vi "Consumer.vi"(8 "error in (no error)":errorcluster, 9 "Data":variant, 10 "Case ID":string, 11 "Scheduler in":refnum<class "Scheduler.lvclass">) -> (0 "error out":errorcluster, 3 "Scheduler out":refnum<class "Scheduler.lvclass">)   [LabVIEW 2020, in "TALOS.lvlib" / "Scheduler.lvlib" / "Scheduler.lvclass"]
uses:
  Scheduler.lvclass
  C:/LabVIEW Code/TALOS/talos/Father of all uServices/Father of all uServices/Father of all uServices.lvclass
  Scheduler Consumer Case Selector.ctl
  Father of all uServices/Father of all uServices/Father of all uServices.lvclass/Father of all uServices.ctl
  Ancestor/Ancestor/Ancestor.lvclass/Ancestor.ctl
  Add RUN Output Data Packet.ctl
  Run Utilities/Schedule Block/Schedule Block.lvclass
  Scheduler.lvclass/Scheduler.ctl
  Run Utilities/Sequence of SBlocks/Sequence of SBlocks.lvclass
  Run Utilities/TypeDefs/Synchronize FPGA Cluster.ctl
  Run Utilities/TypeDefs/Messages/Schedule Message - Standard.ctl
  Run Utilities/Schedule/Schedule.lvclass
  Run Utilities/TypeDefs/Messages/Schedule Message - Parallel.ctl
  Guardian/Guardian Messages/Message to uService Msg/Message to uService Msg.lvclass/Message to uService Msg.ctl
  Father of all uServices/Father of all uServices Messages/Consumer Msg/Consumer Msg.lvclass/Consumer Msg.ctl
  Selection.ctl
  cc9169f9-c1ee-4f38-a286-790ff9248fc5.vi
  Support VIs/Generate Error.vi
  Guardian/Guardian Messages/Message to uService Msg/Send Message to uService.vi
  FGV/Error Memory/Get Error Description.vi
  Support VIs/Get PC name.vi
  Ancestor/Ancestor/Read ID.vi
  Support VIs/Get Class Name.vi
  FGV/Error Memory/Error Memory Core.vi
  <vilib>/AdvancedString/Delimited String to 1D String Array.vi
  Support VIs/Circus Root Path.vi
  FGV/Error Memory/Error Crt Lvl checker.vi
  FGV/Error Memory/Error Memory Core.vi/40c8088d-b597-4017-91af-faa98e00292e.vi
  FGV/Error Memory/Error Memory Core.vi/d4a3ab98-063c-4e44-b43d-fbdcfe6c2be2.vi
  Father of all uServices/Father of all uServices/Father of all uServices.lvclass
  C:/LabVIEW Code/TALOS/builds/Actor Framework PPL/Actor Framework.lvlibp/1abvi3w/vi.lib/ActorFramework/Actor/Actor.lvclass
  Support VIs/Global Memory.vi
  <vilib>/Utility/LVClass/Get LV Class Name.vi
  Support VIs/Is in Packed Library.vi
  Support VIs/TALOS Root path.vi
  Support VIs/Read CSV worksheet.vi
  Support VIs/Global Constants.vi
  <vilib>/Utility/error.llb/General Error Handler.vi
  Support VIs/Error Log.vi
  Add RUN Window.vi
  Father of all uServices/Father of all uServices/Children Methods/Get GUI Item Value - Variant.vi
  builds/Actor Framework PPL/Actor Framework.lvlibp/1abvi3w/vi.lib/ActorFramework/Actor/Read Caller Enqueuer.vi
  builds/Actor Framework PPL/Actor Framework.lvlibp/1abvi3w/vi.lib/ActorFramework/Message Enqueuer/Enqueue.vi
  builds/Actor Framework PPL/Actor Framework.lvlibp/1abvi3w/vi.lib/ActorFramework/Actor/Read Self Enqueuer.vi
  <userlib>/_OpenG.lib/lvdata/lvdata.llb/Get Strings from Enum__ogtk.vi
  Ancestor/Ancestor/Ancestor.lvclass
  <vilib>/Comparison/Equal/Equal Functor/Equal Functor.lvclass
  Guardian/Guardian Messages/Message to uService Msg/Message to uService Msg.lvclass
  Father of all uServices/Father of all uServices Messages/Consumer Msg/Consumer Msg.lvclass
  Scheduler.lvlib
  C:/LabVIEW Code/TALOS/talos/Ancestor/Ancestor/Ancestor.lvclass
  C:/LabVIEW Code/TALOS/talos/Internal uServices/CIRCUS uServices/Scheduler/Scheduler.lvclass
  Run Utilities/Run Utilities.lvlib
  TALOS.lvlib
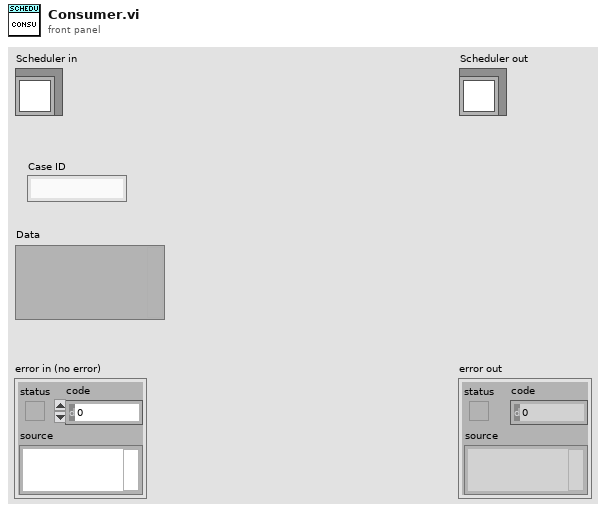
[diagram p1: front panel]
types:
  T1 = typedef "TALOS.lvlib/Scheduler.lvlib/Scheduler.lvclass/Scheduler Consumer Case Selector.ctl" = enum16{"Add SBlock", "Update GUI", "Move SBlock", "Select SBlock", "Update Cont.", "Load", "Save", "Reset", "Send to Tamer", "Edit SBlock", "Duplicate SBlock", "Delete SBlock", "Update SBlock", "Init", "Split/Combine Schedules", "Reschedule", "Load Parameters"}
  T2 = enum8{"Enabled", "Disabled", "Disabled and Grayed Out"}
  T3 = typedef "TALOS.lvlib/Scheduler.lvlib/Scheduler.lvclass/Add RUN Output Data Packet.ctl" = cluster{"Index":i32, "Schedule Block":refnum<class "Schedule Block.lvclass">}
  T4 = enum32{"Invalid", "Standard", "Closed", "Hidden", "Minimized", "Maximized"}
  T5 = typedef "TALOS.lvlib/Run Utilities.lvlib/Schedule Message - Standard.ctl" = cluster{"Schedules":refnum<class "Schedule.lvclass">[]}
  T6 = typedef "TALOS.lvlib/Run Utilities.lvlib/Schedule Message - Parallel.ctl" = cluster{"Schedules":refnum<class "Schedule.lvclass">[], "Synchronised":T7[]}
  T7 = typedef "TALOS.lvlib/Run Utilities.lvlib/Synchronize FPGA Cluster.ctl" = cluster{"Status":bool, "FPGA Name":string}
  T8 = typedef "TALOS.lvlib/Scheduler.lvlib/Scheduler.lvclass/Selection.ctl" = cluster{"Row":i32, "Column":i32}
  T9 = typedef "TALOS.lvlib/Run Utilities.lvlib/Sequence of SBlocks.lvclass/Sequence of SBlcoks - GUI.ctl" = cluster{"Total number of scripts":i32, "Time":string, "Sequence of SBlocks":T10[], "Continuous":bool}
  T10 = typedef "TALOS.lvlib/Run Utilities.lvlib/Schedule Block.lvclass/Schedule Block - simplified GUI.ctl" = cluster{"Bcg Color":u32, "Index":i32, "No. of runs":i32, "Script name":string, "FPGA name":string, "Parameters":string, "Repetitions":i32}
  T11 = cluster{"SBlock Index":i32, "Sequence Index":i32}
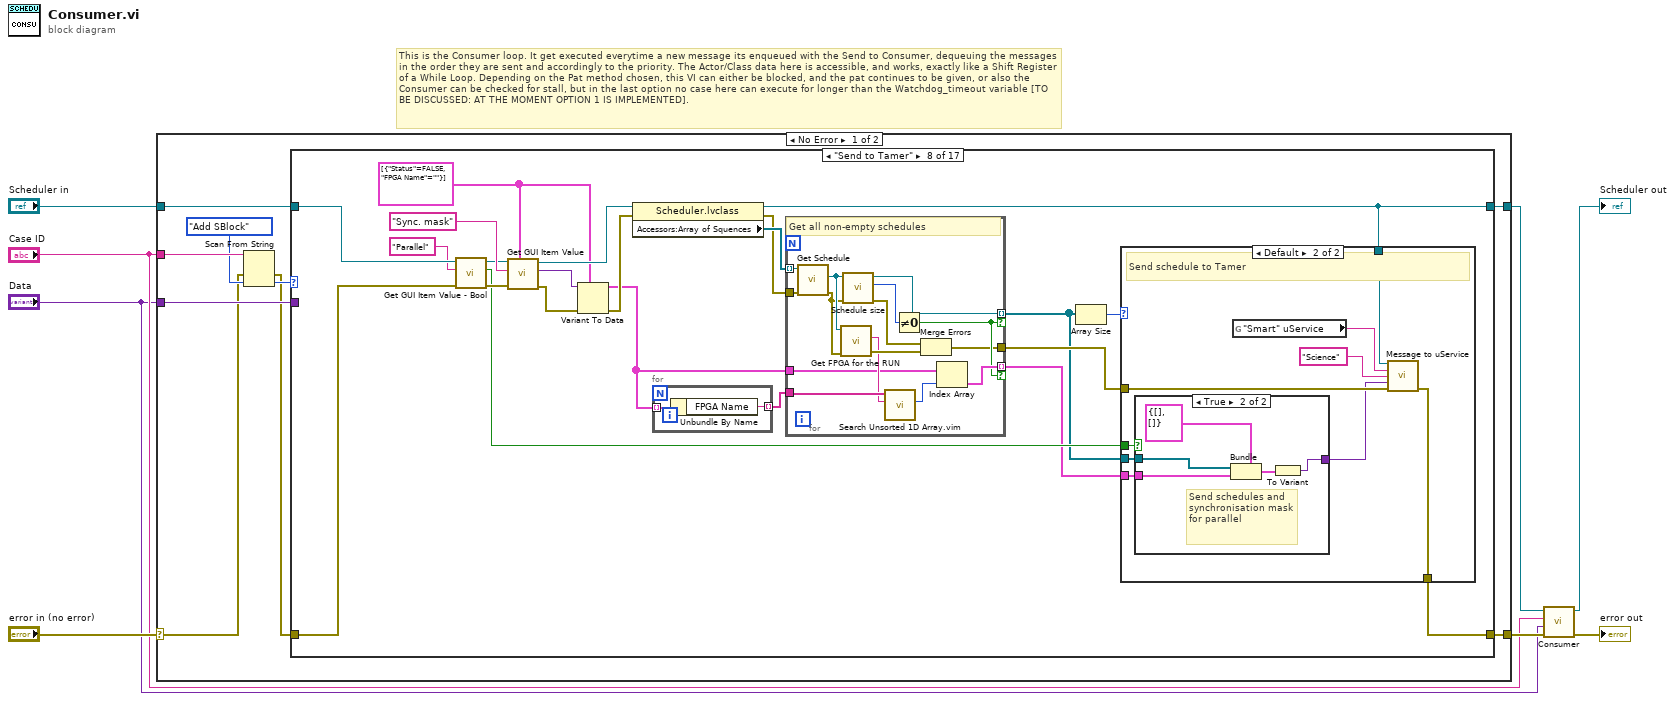
[diagram p0: block diagram]
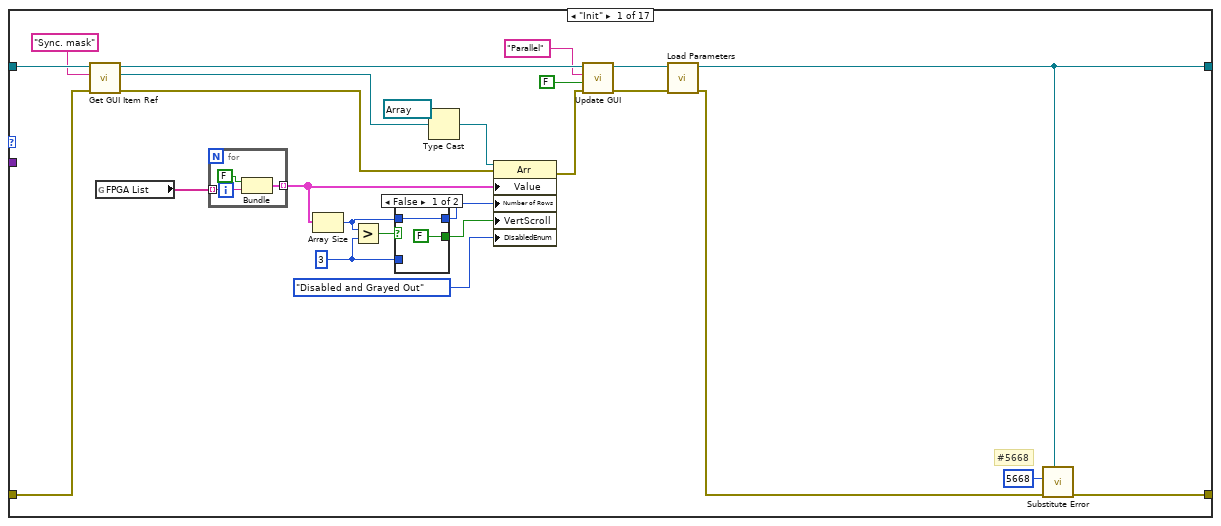
[diagram p2: hidden frame]
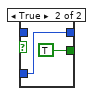
[diagram p3: hidden frame]
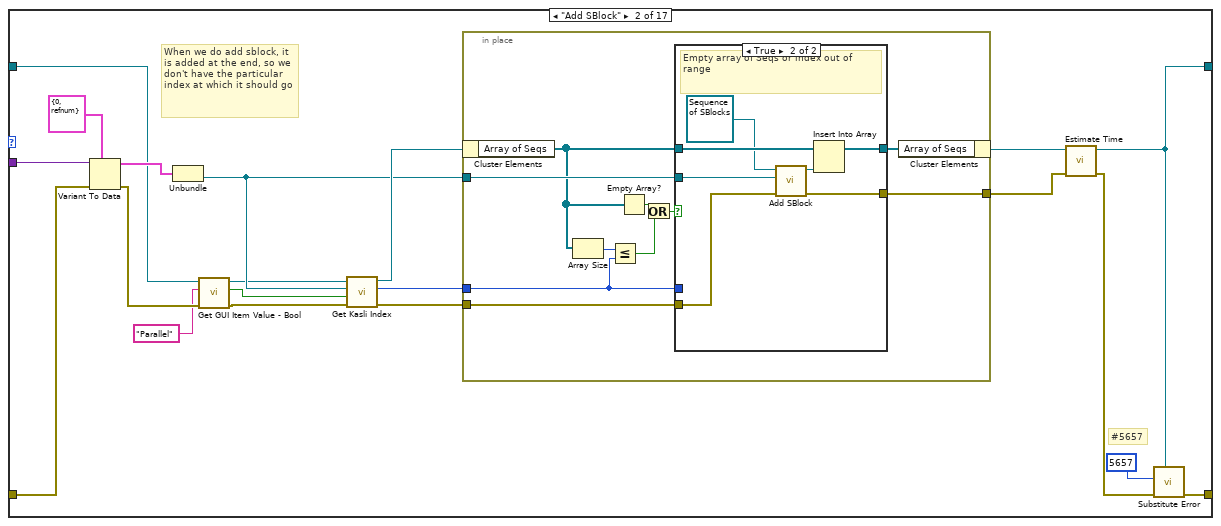
[diagram p4: hidden frame]
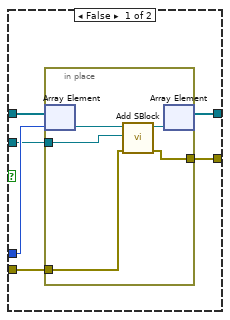
[diagram p5: hidden frame]
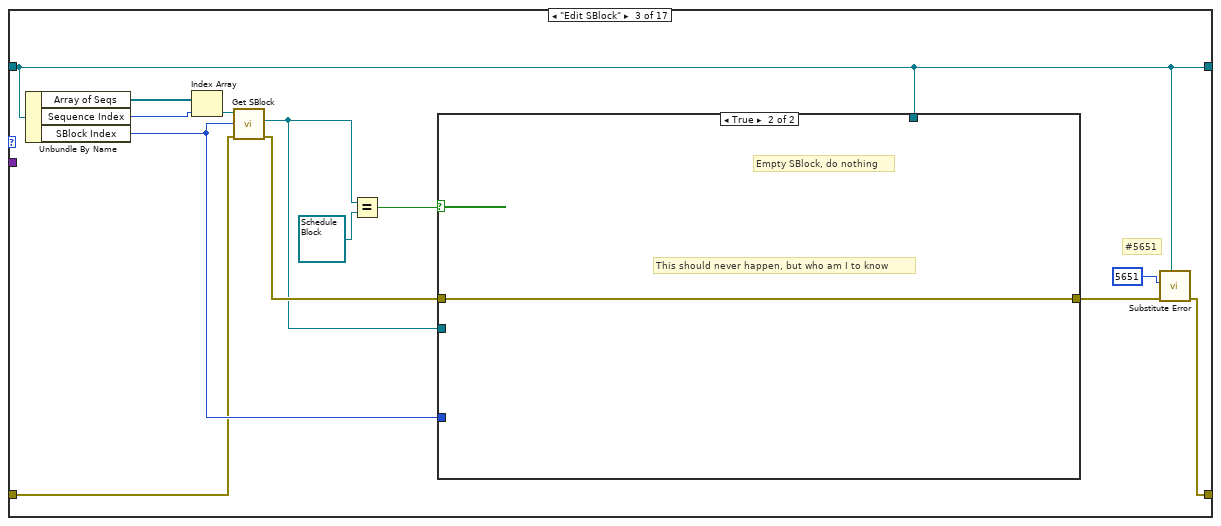
[diagram p6: hidden frame]
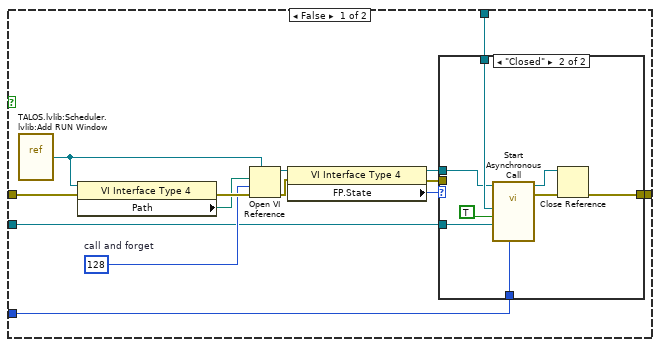
[diagram p7: hidden frame]
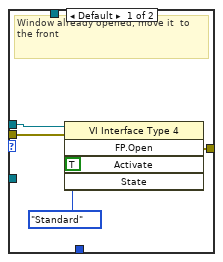
[diagram p8: hidden frame]
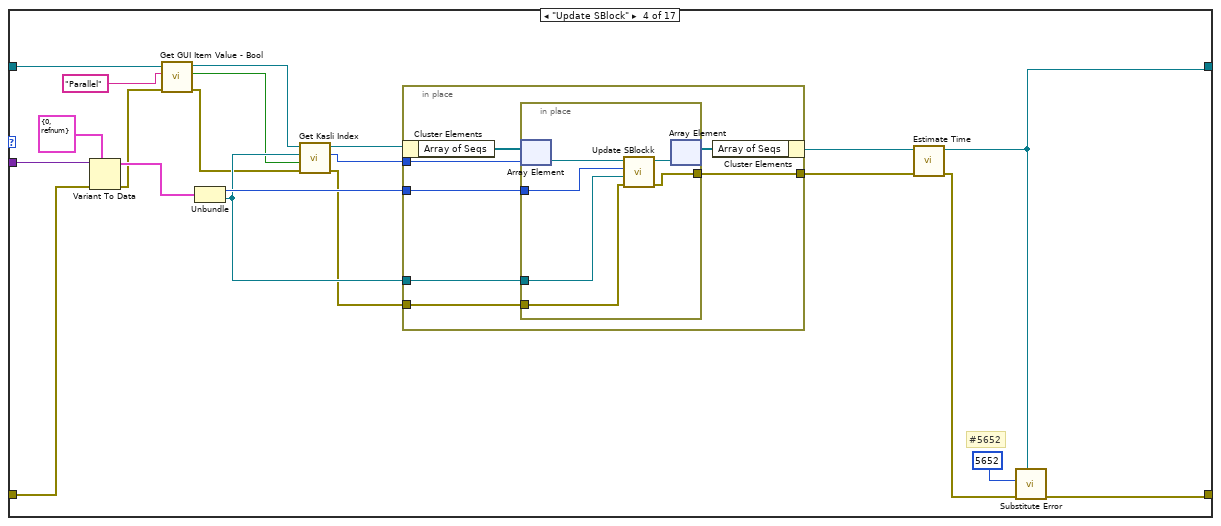
[diagram p9: hidden frame]
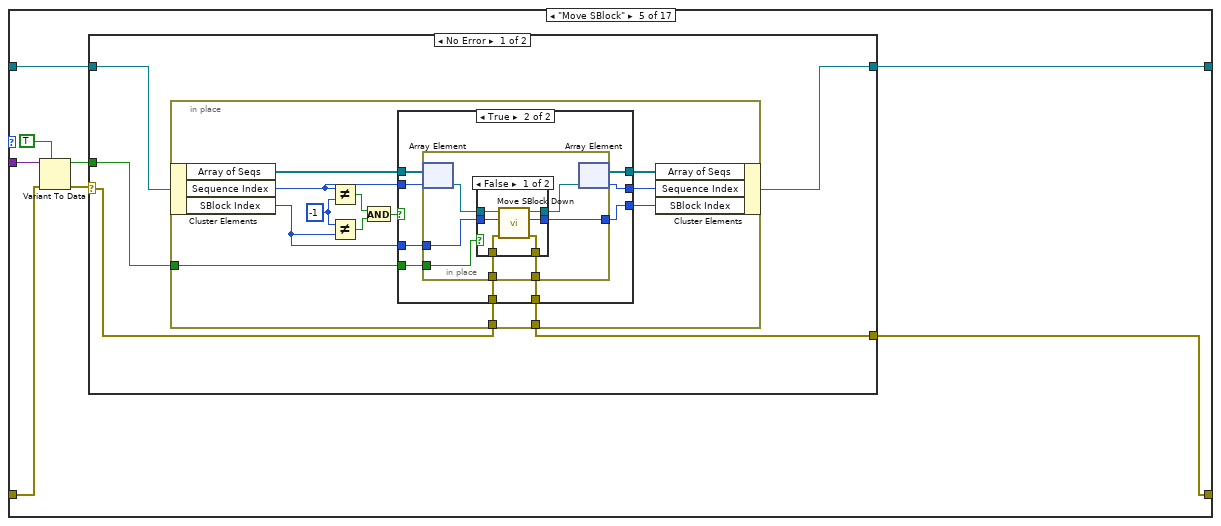
[diagram p10: hidden frame]
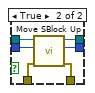
[diagram p12: hidden frame]
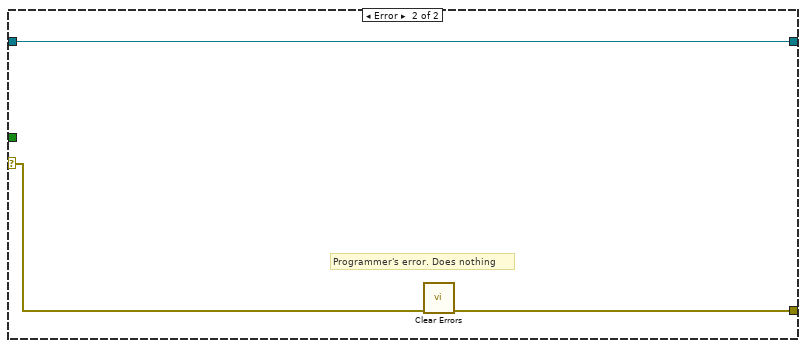
[diagram p13: hidden frame]
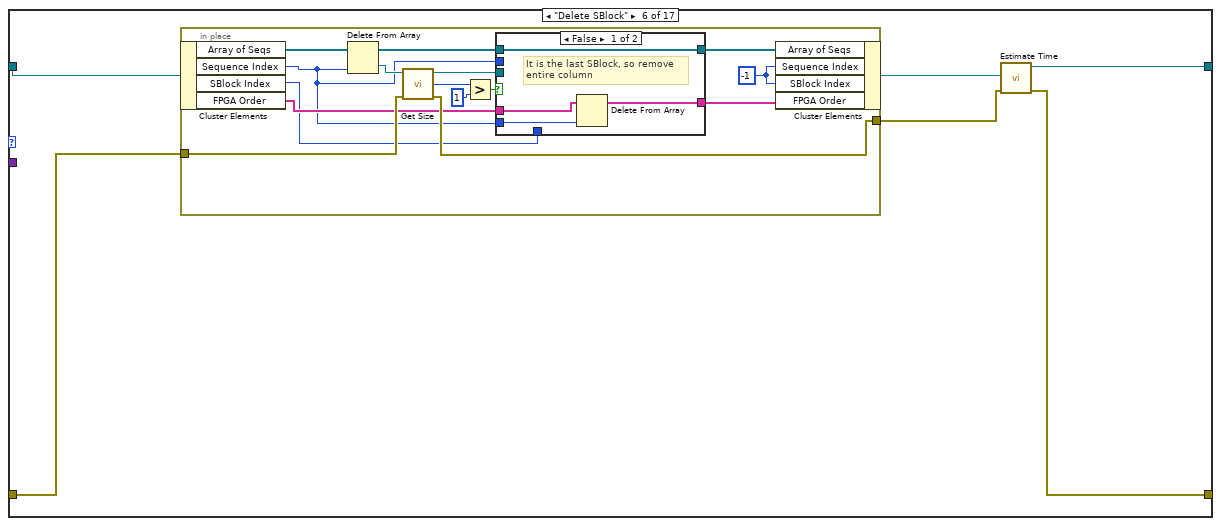
[diagram p14: hidden frame]
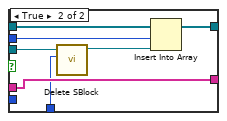
[diagram p15: hidden frame]
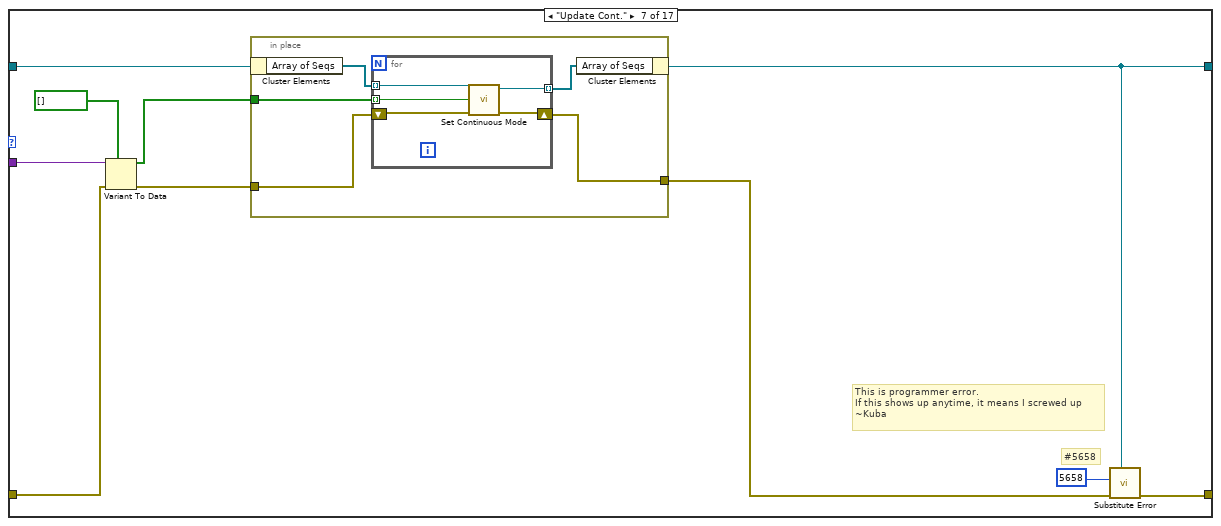
[diagram p16: hidden frame]
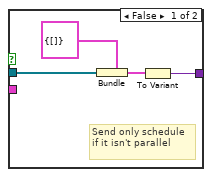
[diagram p18: hidden frame]
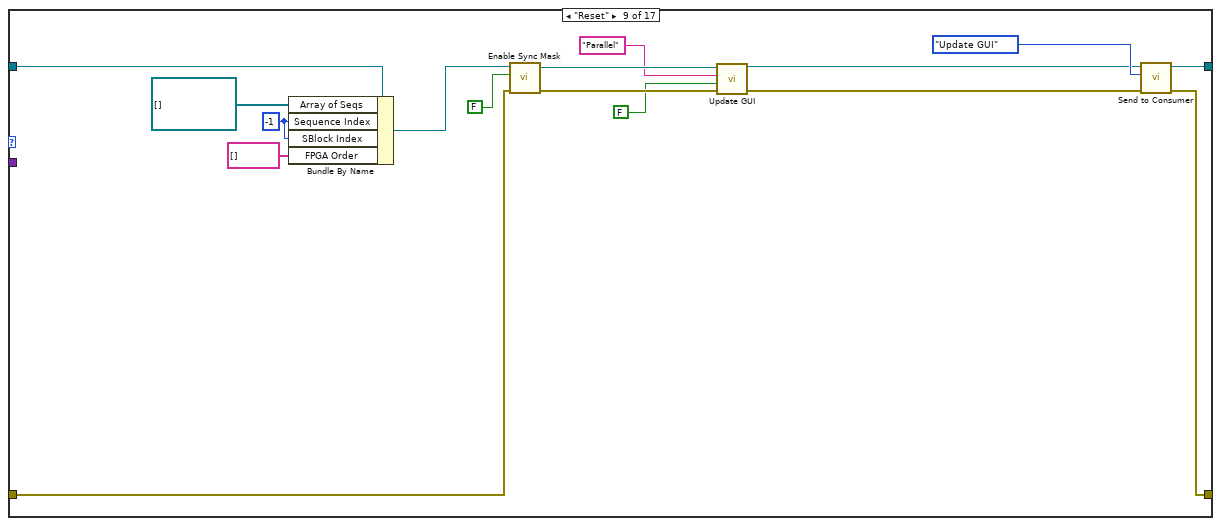
[diagram p19: hidden frame]
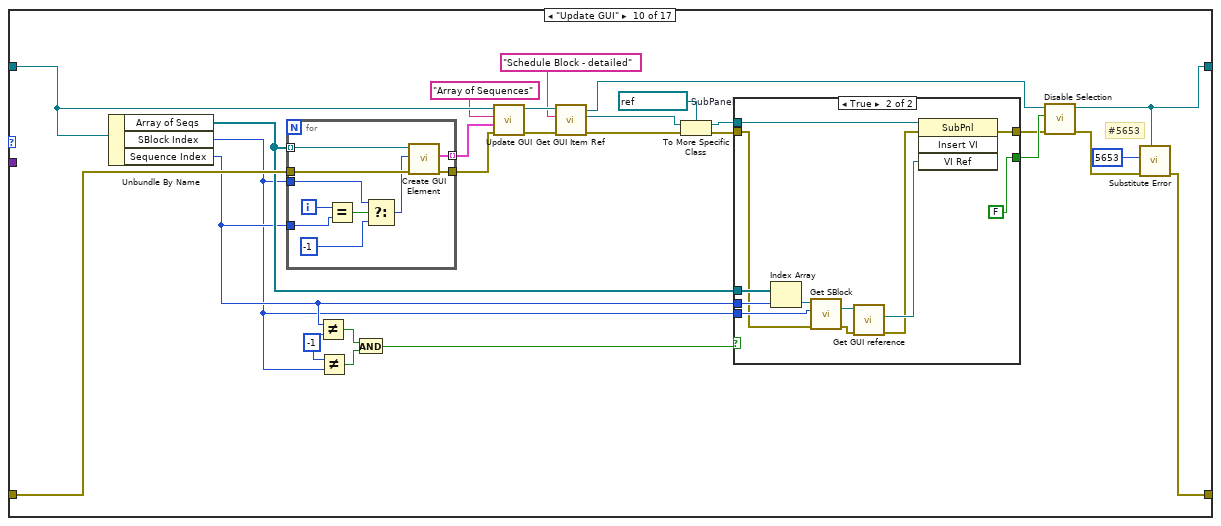
[diagram p20: hidden frame]
diagram:
  # "This is the Consumer loop. It get executed everytime a new message its enqueued with the Send to Consumer, dequeuing the messages in the order they are sent and accordingly to the priority. The Actor/Class data here is accessible, and works, exactly like a Shift Register of a While Loop. Depending on the Pat method chosen, this VI can either be blocked, and the pat continues to be given, or also the Consumer can be checked for stall, but in the last option no case here can execute for longer than the Watchdog_timeout variable [TO BE DISCUSSED: AT THE MOMENT OPTION 1 IS IMPLEMENTED]."
  n1 = case shown="No Error" "error in (no error)" {
    selector: "error in (no error)" -> [w11 w602]
    tunnel: [w10 w603] -> w3
    tunnel: "Scheduler in" -> [w17 w603]
    tunnel: [w15 w602] -> w6
    tunnel: "Case ID" -> [w14 _]
    tunnel: "Data" -> [w16 _]
    frame No Error {
      n2 = Scan From String(input string=w14, error in=w11, default 1=Scheduler_Consumer_Case_Selector."Add SBlock" ("Consumer Case Selector")) -> (error out=w9:errorcluster, output 1=w12:T1)  [unwired: 2 in, 2 out]
      n3 = case shown="\"Send to Tamer\"" w12 {
        tunnel: w17 -> [w35 w55 w108 w143 w180 w239 w275 w301 w350 w384 w416 w468 w496 w519 w565 w595 w600]
        tunnel: w16 -> [_ w69 _ w159 w178 _ w274 _ _ _ w414 w467 _ w518 w567 w597 _]
        tunnel: [w20 w61 w110 w150 w173 w235 w270 w306 w358 w386 w418 w470 w490 w511 w564 w588 w598] -> w15
        tunnel: w9 -> [w34 w66 w103 w155 w174 w238 w273 w300 w347 w383 w413 w466 w497 w516 w566 w592 w601]
        tunnel: [w19 w58 w108 w147 w179 w236 w269 w305 w359 w373 w417 w469 w491 w515 w562 w589 w599] -> w10
        frame "Init" {
          w37 = 3 ("y")
          # "#5668"
          n4 = call "Get GUI Item Ref.vi"("error in (no error)"=w34, "FP Item Name"="Sync. mask", "uService Template in"=w35) -> ("error out"=w29:errorcluster, "Ctl Refnum"=w33:refnum<vi>, "uService Template out"=w28:refnum<class "Scheduler.lvclass">)  [unwired: 6 in]
          n5 = global read "Global Memory.vi" "FPGA List"() -> (w22:string[])
          n6 = for {
            tunnel: w22 -> [w48] mode=indexing
            tunnel: [w47] -> w36 mode=indexing
            n7 = Bundle(FALSE, "AEgIS PCs List"=w48) -> (w47:cluster{bool, "AEgIS PCs List":string})  [unwired: 1 in]
          }
          n8 = Array Size(array=w36) -> (size(s)=w39:i32)
          n9 = Greater?(x=w39, y=w37) -> (0:w42:bool)
          n10 = case shown="False" w42 {
            tunnel: [w43 w45] -> w41
            tunnel: [FALSE TRUE] -> w40
            tunnel: w39 -> [w43 _]
            tunnel: w37 -> [_ w45]
            frame False {
            }
            frame True {
            }
          }
          n11 = Type Cast(type=refnum<vi> refnum ("reference"), x=w33) -> (*(type *) &x=w31:refnum<vi>)
          n12 = property class="Arr"(reference=w31, error in=w29, "Value"=w36, "Number of Rows"=w41, "VertScroll"=w40, "DisabledEnum"=T2."Disabled and Grayed Out" ("Disabled")) -> (error out=w27:errorcluster)  [unwired: 1 out]
          n13 = call "Update GUI.vi"("error in (no error)"=w27, "Data"=FALSE, "GUI Item Name"="Parallel", "uService Template in"=w28) -> ("error out"=w24:errorcluster, "uService Template out"=w23:refnum<class "Scheduler.lvclass">)  [unwired: 6 in]
          n14 = call-dynamic "Load Parameters.vi"("error in (no error)"=w24, "Scheduler in"=w23) -> ("error out"=w21:errorcluster, "Scheduler out"=w19:refnum<class "Scheduler.lvclass">)  [unwired: 8 in]
          n15 = call "Substitute Error.vi"("LabVIEW Object"=w19, "error in (no error)"=w21, "Error Code"=5668) -> ("error out"=w20:errorcluster)  [unwired: 8 in]
        }
        frame "Add SBlock" {
          # "When we do add sblock, it is added at the end, so we don't have the particular index at which it should go"
          # "#5657"
          n16 = Variant To Data(error in=w66, type=T3 {"Index"=0, "Schedule Block"=refnum} ("Cluster"), Variant=w69) -> (data=w67:T3, error out=w54:errorcluster)
          n17 = Unbundle(w67) -> ("Schedule Block"=w62:refnum<class "Schedule Block.lvclass">)  [unwired: 1 out]
          n18 = call "Get GUI Item Value - Bool.vi"("error in (no error)"=w54, "FP Item Name"="Parallel", "uService Template in"=w55) -> ("error out"=w53:errorcluster, "Value"=w51:bool, "uService Template out"=w52:refnum<class "Scheduler.lvclass">)  [unwired: 6 in]
          n19 = call-dynamic "Get Kasli Index.vi"("error in (no error)"=w53, "Parallel?"=w51, "Schedule Block"=w62, "Scheduler in"=w52) -> ("error out"=w63:errorcluster, "Index"=w64:i32, "Scheduler out"=w65:refnum<class "Scheduler.lvclass">)  [unwired: 5 in]
          n20 = in-place {
            in-place-border: w64 -> [w73]
            in-place-border: w62 -> [w79]
            in-place-border: w63 -> [w77]
            in-place-border: [w76] -> w56
            n21 = in-place-cluster #1(w65) -> ("Array of Seqs"=w71:refnum<class "Sequence of SBlocks.lvclass">[])
            n22 = Array Size(array=w71) -> (size(s)=w74:i32)
            n23 = Less Or Equal?(x=w74, y=w73) -> (x <= y?=w72:bool)
            n24 = Empty Array?(array=w71) -> (empty?=w75:bool)
            n25 = Or(x=w75, y=w72) -> (x .or. y?=w70:bool)
            n26 = case shown="True" w70 {
              tunnel: w73 -> [w85 _]
              tunnel: w71 -> [w84 w97]
              tunnel: w79 -> [w83 w94]
              tunnel: [w82 w96] -> w78
              tunnel: w77 -> [w81 w92]
              tunnel: [w80 w91] -> w76
              frame False {
                n27 = in-place {
                  in-place-border: w83 -> [w87]
                  in-place-border: w81 -> [w88]
                  in-place-border: [w86] -> w80
                  n28 = in-place-array #2(w84, w85) -> (w90:refnum<class "Sequence of SBlocks.lvclass">)
                  n29 = call-dynamic "Add SBlock.vi"("error in (no error)"=w88, "new SBlock"=w87, "Sequence of SBlocks in"=w90) -> ("error out"=w86:errorcluster, "Sequence of SBlocks out"=w89:refnum<class "Sequence of SBlocks.lvclass">)  [unwired: 7 in]
                  n30 = in-place-array #2(w89) -> (w82:refnum<class "Sequence of SBlocks.lvclass">[])  [unwired: 1 out]
                }
              }
              frame True {
                # "Empty array of Seqs or index out of range"
                n31 = call-dynamic "Add SBlock.vi"("error in (no error)"=w92, "new SBlock"=w94, "Sequence of SBlocks in"=refnum<class "Sequence of SBlocks.lvclass"> refnum ("new element/subarray")) -> ("error out"=w91:errorcluster, "Sequence of SBlocks out"=w93:refnum<class "Sequence of SBlocks.lvclass">)  [unwired: 7 in]
                n32 = Insert Into Array(array=w97, new element=w93) -> (w96:refnum<class "Sequence of SBlocks.lvclass">[])  [unwired: 1 in]
              }
            }
            n33 = in-place-cluster #1("Array of Seqs"=w78) -> (w59:refnum<class "Scheduler.lvclass">)
          }
          n34 = call-dynamic "Estimate Time.vi"("error in (no error)"=w56, "Scheduler in"=w59) -> ("error out"=w57:errorcluster, "Scheduler out"=w58:refnum<class "Scheduler.lvclass">)  [unwired: 8 in]
          n35 = call "Substitute Error.vi"("LabVIEW Object"=w58, "error in (no error)"=w57, "Error Code"=5657) -> ("error out"=w61:errorcluster)  [unwired: 8 in]
        }
        frame "Edit SBlock" {
          # "#5651"
          n36 = Unbundle By Name(w108) -> ("Array of Seqs"=w106:refnum<class "Sequence of SBlocks.lvclass">[], "Sequence Index"=w105:i32, "SBlock Index"=w104:i32)
          n37 = Index Array(array=w106, index=w105) -> (element=w102:refnum<class "Sequence of SBlocks.lvclass">)
          n38 = call-dynamic "Get SBlock.vi"("error in (no error)"=w103, "index"=w104, "Sequence of SBlocks in"=w102) -> ("error out"=w101:errorcluster, "Schedule Block"=w98:refnum<class "Schedule Block.lvclass">)  [unwired: 6 in, 1 out]
          n39 = Equal?(x=w98, y=refnum<class "Schedule Block.lvclass"> refnum) -> (x = y?=w99:bool)
          n40 = case shown="True" w99 {
            tunnel: w108 -> [w123 _]
            tunnel: [w122 w138] -> w107
            tunnel: w101 -> [w121 w138]
            tunnel: w104 -> [w120 _]
            tunnel: w98 -> [w115 _]
            frame False {
              w118 = 128  # call and forget
              n41 = vi-ref "TALOS.lvlib:Scheduler.lvlib:Add RUN Window.vi"() -> (w117:refnum<vi>)
              n42 = property class="VI Interface Type 4"(reference=w117, error in=w121) -> (error out=w124:errorcluster, "Path"=w116:path)  [unwired: 1 out]
              n43 = Open VI Reference(type specifier VI Refnum (for type only)=w117, vi path=w116, options=w118, error in (no error)=w124) -> (vi reference=w119:refnum<vi>, error out=w114:errorcluster)  [unwired: 2 in]
              n44 = property class="VI Interface Type 4"(reference=w119, error in=w114) -> (reference out=w112:refnum<vi>, error out=w111:errorcluster, "FP.State"=w113:T4)
              n45 = case shown="\"Closed\"" w113 {
                tunnel: w123 -> [_ w137]
                tunnel: [w126 w136] -> w122
                tunnel: w120 -> [_ w135]
                tunnel: w115 -> [_ w131]
                tunnel: w112 -> [w125 w130]
                tunnel: w111 -> [w127 _]
                frame Default {
                  # "Window already opened, move it  to the front"
                  n46 = invoke class="VI Interface Type 4" method="FP.Open"(reference=w125, error in=w127, "Activate"=TRUE ("Activate?"), "State"=T4."Standard") -> (error out=w126:errorcluster)  [unwired: 1 in, 4 out]
                }
                frame "Closed" {
                  n47 = call-by-ref "Start Asynchronous Call"(reference=w130, "Index"=w135, "Schedule Block"=w131, "Modify"=TRUE, "Scheduler in"=w137) -> (reference out=w133:refnum<vi>, error out=w134:errorcluster)  [unwired: 7 in, 2 out]
                  n48 = Close Reference(reference=w133, error in (no error)=w134) -> (error out=w136:errorcluster)
                }
              }
            }
            frame True {
              # "This should never happen, but who am I to know"
              # "Empty SBlock, do nothing"
            }
          }
          n49 = call "Substitute Error.vi"("LabVIEW Object"=w108, "error in (no error)"=w107, "Error Code"=5651) -> ("error out"=w110:errorcluster)  [unwired: 8 in]
        }
        frame "Update SBlock" {
          # "#5652"
          n50 = Variant To Data(error in=w155, type=T3 {"Index"=0, "Schedule Block"=refnum} ("Cluster"), Variant=w159) -> (data=w157:T3, error out=w141:errorcluster)
          n51 = call "Get GUI Item Value - Bool.vi"("error in (no error)"=w141, "FP Item Name"="Parallel", "uService Template in"=w143) -> ("error out"=w140:errorcluster, "Value"=w139:bool, "uService Template out"=w142:refnum<class "Scheduler.lvclass">)  [unwired: 6 in]
          n52 = Unbundle(w157) -> ("Index"=w156:i32, "Schedule Block"=w152:refnum<class "Schedule Block.lvclass">)
          n53 = call-dynamic "Get Kasli Index.vi"("error in (no error)"=w140, "Parallel?"=w139, "Schedule Block"=w152, "Scheduler in"=w142) -> ("error out"=w151:errorcluster, "Index"=w153:i32, "Scheduler out"=w154:refnum<class "Scheduler.lvclass">)  [unwired: 5 in]
          n54 = in-place {
            in-place-border: w156 -> [w162]
            in-place-border: w152 -> [w165]
            in-place-border: w151 -> [w163]
            in-place-border: w153 -> [w161]
            in-place-border: [w160] -> w146
            n55 = in-place-cluster #3(w154) -> ("Array of Seqs"=w166:refnum<class "Sequence of SBlocks.lvclass">[])
            n56 = in-place {
              in-place-border: w165 -> [w171]
              in-place-border: w163 -> [w169]
              in-place-border: w162 -> [w170]
              in-place-border: [w167] -> w160
              n57 = in-place-array #4(w166, w161) -> (w172:refnum<class "Sequence of SBlocks.lvclass">)
              n58 = call-dynamic "Update SBlockk.vi"("error in (no error)"=w169, "element"=w171, "Index"=w170, "Sequence of SBlocks in"=w172) -> ("error out"=w167:errorcluster, "Sequence of SBlocks out"=w168:refnum<class "Sequence of SBlocks.lvclass">)  [unwired: 6 in]
              n59 = in-place-array #4(w168) -> (w164:refnum<class "Sequence of SBlocks.lvclass">[])  [unwired: 1 out]
            }
            n60 = in-place-cluster #3("Array of Seqs"=w164) -> (w148:refnum<class "Scheduler.lvclass">)
          }
          n61 = call-dynamic "Estimate Time.vi"("error in (no error)"=w146, "Scheduler in"=w148) -> ("error out"=w145:errorcluster, "Scheduler out"=w147:refnum<class "Scheduler.lvclass">)  [unwired: 8 in]
          n62 = call "Substitute Error.vi"("LabVIEW Object"=w147, "error in (no error)"=w145, "Error Code"=5652) -> ("error out"=w150:errorcluster)  [unwired: 8 in]
        }
        frame "Move SBlock" {
          n63 = Variant To Data(error in=w174, type=TRUE, Variant=w178) -> (data=w176:bool, error out=w175:errorcluster)
          n64 = case shown="No Error" w175 {
            selector: w175 -> [w182 w232]
            tunnel: w180 -> [w185 w233]
            tunnel: [w184 w233] -> w179
            tunnel: w176 -> [w183 _]
            tunnel: [w181 w231] -> w173
            frame No Error {
              n65 = in-place {
                in-place-border: w182 -> [w194]
                in-place-border: [w193] -> w181
                in-place-border: w183 -> [w186]
                w198 = -1 ("y")
                n66 = in-place-cluster #5(w185) -> ("Array of Seqs"=w192:refnum<class "Sequence of SBlocks.lvclass">[], "Sequence Index"=w191:i32, "SBlock Index"=w190:i32)
                n67 = Not Equal?(x=w191, y=w198) -> (x != y?=w196:bool)
                n68 = Not Equal?(x=w198, y=w190) -> (x != y?=w197:bool)
                n69 = And(x=w196, y=w197) -> (x .and. y?=w195:bool)
                n70 = case shown="True" w195 {
                  tunnel: w192 -> [w199 w211]
                  tunnel: w191 -> [w200 w210]
                  tunnel: w190 -> [w201 w209]
                  tunnel: w194 -> [w202 w208]
                  tunnel: [w202 w207] -> w193
                  tunnel: [w199 w206] -> w189
                  tunnel: [w200 w205] -> w188
                  tunnel: [w201 w204] -> w187
                  tunnel: w186 -> [_ w203]
                  frame False {
                  }
                  frame True {
                    n71 = in-place {
                      in-place-border: w209 -> [w217]
                      in-place-border: w208 -> [w216]
                      in-place-border: [w214] -> w204
                      in-place-border: [w213] -> w207
                      in-place-border: w203 -> [w212]
                      n72 = in-place-array #6(w211, w210) -> (w218:refnum<class "Sequence of SBlocks.lvclass">)
                      n73 = case shown="False" w212 {
                        tunnel: w218 -> [w224 w230]
                        tunnel: w217 -> [w223 w229]
                        tunnel: w216 -> [w222 w228]
                        tunnel: [w219 w227] -> w215
                        tunnel: [w220 w226] -> w214
                        tunnel: [w221 w225] -> w213
                        frame False {
                          n74 = call-dynamic "Move SBlock Down.vi"("error in (no error)"=w222, "index"=w223, "Sequence of SBlocks in"=w224) -> ("error out"=w221:errorcluster, "New Index"=w220:i32, "Sequence of SBlocks out"=w219:refnum<class "Sequence of SBlocks.lvclass">)  [unwired: 6 in]
                        }
                        frame True {
                          n75 = call-dynamic "Move SBlock Up.vi"("error in (no error)"=w228, "index"=w229, "Sequence of SBlocks in"=w230) -> ("error out"=w225:errorcluster, "New Index"=w226:i32, "Sequence of SBlocks out"=w227:refnum<class "Sequence of SBlocks.lvclass">)  [unwired: 6 in]
                        }
                      }
                      n76 = in-place-array #6(w215) -> (w206:refnum<class "Sequence of SBlocks.lvclass">[], w205:i32)
                    }
                  }
                }
                n77 = in-place-cluster #5("Array of Seqs"=w189, "Sequence Index"=w188, "SBlock Index"=w187) -> (w184:refnum<class "Scheduler.lvclass">)
              }
            }
            frame Error {
              # "Programmer's error. Does nothing"
              n78 = call <vilib>:"Clear Errors.vi"("error in (no error)"=w232) -> ("error out"=w231:errorcluster)  [unwired: 5 in, 1 out]
            }
          }
        }
        frame "Delete SBlock" {
          n79 = in-place {
            in-place-border: w238 -> [w251]
            in-place-border: [w246] -> w234
            w254 = -1 ("Sequence Index")
            n80 = in-place-cluster #7(w239) -> ("Array of Seqs"=w253:refnum<class "Sequence of SBlocks.lvclass">[], "Sequence Index"=w242:i32, "SBlock Index"=w241:i32, "FPGA Order"=w244:string[])
            n81 = Delete From Array(array=w253, index=w242) -> (deleted portion=w245:refnum<class "Sequence of SBlocks.lvclass">, array with subset deleted=w240:refnum<class "Sequence of SBlocks.lvclass">[])  [unwired: 1 in]
            n82 = call-dynamic "Get Size.vi"("error in (no error)"=w251, "Sequence of SBlocks in"=w245) -> ("error out"=w246:errorcluster, "size"=w250:i32, "Sequence of SBlocks out"=w252:refnum<class "Sequence of SBlocks.lvclass">)  [unwired: 7 in]
            n83 = Greater?(x=w250, y=1) -> (0:w247:bool)
            n84 = case shown="False" w247 {
              tunnel: w240 -> [w258 w265]
              tunnel: w252 -> [_ w261]
              tunnel: w242 -> [_ w264]
              tunnel: [w258 w263] -> w248
              tunnel: w244 -> [w257 w262]
              tunnel: w242 -> [w256 _]
              tunnel: [w255 w262] -> w243
              tunnel: w241 -> [_ w260]
              frame False {
                # "It is the last SBlock, so remove entire column"
                n85 = Delete From Array(array=w257, index=w256) -> (array with subset deleted=w255:string[])  [unwired: 1 in, 1 out]
              }
              frame True {
                n86 = call-dynamic "Delete SBlock.vi"("index"=w260, "Sequence of SBlocks in"=w261) -> ("Sequence of SBlocks out"=w259:refnum<class "Sequence of SBlocks.lvclass">)  [unwired: 7 in, 2 out]
                n87 = Insert Into Array(array=w265, index=w264, new element=w259) -> (w263:refnum<class "Sequence of SBlocks.lvclass">[])
              }
            }
            n88 = in-place-cluster #7("Array of Seqs"=w248, "Sequence Index"=w254, "SBlock Index"=w254, "FPGA Order"=w243) -> (w237:refnum<class "Scheduler.lvclass">)
          }
          n89 = call-dynamic "Estimate Time.vi"("error in (no error)"=w234, "Scheduler in"=w237) -> ("error out"=w235:errorcluster, "Scheduler out"=w236:refnum<class "Scheduler.lvclass">)  [unwired: 8 in]
        }
        frame "Update Cont." {
          # "This is programmer error.\nIf this shows up anytime, it means I screwed up\n~Kuba"
          # "#5658"
          n90 = Variant To Data(error in=w273, type=bool[] [], Variant=w274) -> (data=w266:bool[], error out=w272:errorcluster)
          n91 = in-place {
            in-place-border: w272 -> [w280]
            in-place-border: [w279] -> w271
            in-place-border: w266 -> [w277]
            n92 = in-place-cluster #8(w275) -> ("Array of Seqs"=w278:refnum<class "Sequence of SBlocks.lvclass">[])
            n93 = for {
              shift-right: [w284] -> w279
              shift-left: w280 -> [w285]
              tunnel: w278 -> [w283] mode=indexing
              tunnel: w277 -> [w282] mode=indexing
              tunnel: [w281] -> w276 mode=indexing
              n94 = call-dynamic "Set Continuous Mode.vi"("error in (no error)"=w285, "Continuous?"=w282, "Sequence of SBlocks in"=w283) -> ("error out"=w284:errorcluster, "Sequence of SBlocks out"=w281:refnum<class "Sequence of SBlocks.lvclass">)  [unwired: 7 in]
            }
            n95 = in-place-cluster #8("Array of Seqs"=w276) -> (w269:refnum<class "Scheduler.lvclass">)
          }
          n96 = call "Substitute Error.vi"("LabVIEW Object"=w269, "error in (no error)"=w271, "Error Code"=5658) -> ("error out"=w270:errorcluster)  [unwired: 8 in]
        }
        frame "Send to Tamer" {
          w286 = T7[] [{"Status"=FALSE, "FPGA Name"=""}]
          n97 = call "Get GUI Item Value - Bool.vi"("error in (no error)"=w300, "FP Item Name"="Parallel", "uService Template in"=w301) -> ("error out"=w298:errorcluster, "Value"=w292:bool, "uService Template out"=w287:refnum<class "Scheduler.lvclass">)  [unwired: 6 in]
          n98 = call-poly "Get GUI Item Value.vi"("Default"=w286, "error in (no error)"=w298, "FP Item Name"="Sync. mask", "uService Template in"=w287) -> ("error out"=w295:errorcluster, "Value"=w296:variant, "uService Template out"=w294:refnum<class "Scheduler.lvclass">)  [unwired: 5 in]
          n99 = Variant To Data(error in=w295, type=w286, Variant=w296) -> (data=w290:T7[], error out=w293:errorcluster)
          n100 = property class="Scheduler.lvclass"(reference=w294, error in=w293) -> (reference out=w305:refnum<class "Scheduler.lvclass">, error out=w303:errorcluster, "Accessors:Array of Squences"=w304:refnum<class "Sequence of SBlocks.lvclass">[])
          n101 = for {
            tunnel: w290 -> [w309] mode=indexing
            tunnel: [w308] -> w289 mode=indexing
            n102 = Unbundle By Name(w309) -> ("FPGA Name"=w308:string)
          }
          n103 = for {
            tunnel: [w310] -> w307
            tunnel: [w321] -> w291 mode=indexing if=w311
            tunnel: w304 -> [w324] mode=indexing
            tunnel: w303 -> [w323]
            tunnel: w290 -> [w314]
            tunnel: w289 -> [w316]
            tunnel: [w312] -> w288 mode=indexing if=w311
            # "Get all non-empty schedules"
            n104 = call-dynamic "Get Schedule.vi"("error in (no error)"=w323, "Sequence of SBlocks in"=w324) -> ("error out"=w319:errorcluster, "Schedule"=w320:refnum<class "Schedule.lvclass">)  [unwired: 7 in, 1 out]
            n105 = call-dynamic "Get FPGA for the RUN.vi"("error in (no error)"=w319, "Schedule in"=w320) -> ("error out"=w317:errorcluster, "FPGA Name"=w315:string)  [unwired: 7 in, 1 out]
            n106 = call-dynamic "Schedule size.vi"("error in (no error)"=w319, "Schedule in"=w320) -> ("error out"=w318:errorcluster, "Size"=w322:i32, "Schedule out"=w321:refnum<class "Schedule.lvclass">)  [unwired: 7 in]
            n107 = call "Search Unsorted 1D Array.vim"("element"=w315, "unsorted 1D array"=w316) -> ("index of element"=w313:i32)  [unwired: 9 in]
            n108 = Not Equal To 0?(x=w322) -> (x != 0?=w311:bool)
            n109 = Merge Errors(w318, w317) -> (w310:errorcluster)
            n110 = Index Array(array=w314, index=w313) -> (element=w312:T7)
          }
          n111 = Array Size(array=w291) -> (size(s)=w302:i32)
          n112 = case shown="Default" w302 {
            tunnel: w305 -> [_ w333]
            tunnel: [w325 w332] -> w306
            tunnel: w307 -> [w325 w331]
            tunnel: w292 -> [_ w330]
            tunnel: w291 -> [_ w329]
            tunnel: w288 -> [_ w326]
            frame 0 {
              # "There are no non-empty schedules, do nothing"
            }
            frame Default {
              # "Send schedule to Tamer"
              n113 = case shown="True" w330 {
                tunnel: w329 -> [w338 w342]
                tunnel: w326 -> [_ w341]
                tunnel: [w335 w339] -> w328
                frame False {
                  # "Send only schedule if it isn't parallel"
                  n114 = Bundle(cluster=T5 {"Schedules"=[]} ("Schedule message - parallel"), "Schedules"=w338) -> (w336:T5)
                  n115 = To Variant(anything=w336) -> (Variant=w335:variant)
                }
                frame True {
                  # "Send schedules and synchronisation mask for parallel"
                  n116 = Bundle(cluster=T6 {"Schedules"=[], "Synchronised"=[]}, "Schedules"=w342, "Synchronised"=w341) -> (w340:T6)
                  n117 = To Variant(anything=w340) -> (Variant=w339:variant)
                }
              }
              n118 = global read "Global Constants.vi" "\"Smart\" uService"() -> (w327:string)
              n119 = call "Message to uService.vi"("Father of all uServices in"=w333, "uService ID"=w327, "Message"="Science", "Data"=w328, "error in (no error)"=w331) -> ("error out"=w332:errorcluster)  [unwired: 9 in, 1 out]
            }
          }
        }
        frame "Reset" {
          w346 = -1 ("Sequence Index")
          n120 = Bundle By Name(cluster=w350, "Array of Seqs"=refnum<class "Sequence of SBlocks.lvclass">[] [] ("Array of Squences"), "Sequence Index"=w346, "SBlock Index"=w346, "FPGA Order"=string[] [] ("Kasli Order")) -> (w348:refnum<class "Scheduler.lvclass">)
          n121 = call-dynamic "Enable Sync Mask.vi"("error in (no error)"=w347, "Enable"=FALSE, "Scheduler in"=w348) -> ("error out"=w356:errorcluster, "Scheduler out"=w355:refnum<class "Scheduler.lvclass">)  [unwired: 7 in]
          n122 = call "Update GUI.vi"("error in (no error)"=w356, "Data"=FALSE, "GUI Item Name"="Parallel", "uService Template in"=w355) -> ("error out"=w354:errorcluster, "uService Template out"=w344:refnum<class "Scheduler.lvclass">)  [unwired: 6 in]
          n123 = call "Send to Consumer.vi"("error in (no error)"=w354, "Case ID"=Scheduler_Consumer_Case_Selector."Update GUI" ("Consumer Case Selector"), "uService Template in"=w344) -> ("error out"=w358:errorcluster, "uService Template out"=w359:refnum<class "Scheduler.lvclass">)  [unwired: 7 in]
        }
        frame "Update GUI" {
          w362 = refnum<vi> refnum  # SubPanel
          w374 = -1 ("y")
          # "#5653"
          n124 = Unbundle By Name(w384) -> ("Array of Seqs"=w380:refnum<class "Sequence of SBlocks.lvclass">[], "SBlock Index"=w375:i32, "Sequence Index"=w376:i32)
          n125 = for {
            tunnel: w380 -> [w412] mode=indexing
            tunnel: w383 -> [w411]
            tunnel: w376 -> [w409]
            tunnel: w375 -> [w407]
            tunnel: [w404] -> w382 mode=indexing
            tunnel: [w403] -> w381
            i -> [w408]
            n126 = Equal?(x=w408, y=w409) -> (x = y?=w410:bool)
            n127 = Select(t=w407, s=w410, f=-1) -> (s? t:f=w405:i32)
            n128 = call-dynamic "Create GUI Element.vi"("error in (no error)"=w411, "Highlight index"=w405, "Sequence of SBlocks in"=w412) -> ("error out"=w403:errorcluster, "Sequence of SBlocks - GUI"=w404:T9)  [unwired: 6 in, 1 out]
          }
          n129 = Not Equal?(x=w376, y=w374) -> (x != y?=w379:bool)
          n130 = Not Equal?(x=w374, y=w375) -> (x != y?=w378:bool)
          n131 = And(x=w379, y=w378) -> (x .and. y?=w377:bool)
          n132 = call "Update GUI.vi"("error in (no error)"=w381, "Data"=w382, "GUI Item Name"="Array of Sequences", "uService Template in"=w384) -> ("error out"=w368:errorcluster, "uService Template out"=w369:refnum<class "Scheduler.lvclass">)  [unwired: 6 in]
          n133 = call "Get GUI Item Ref.vi"("error in (no error)"=w368, "FP Item Name"="Schedule Block - detailed", "uService Template in"=w369) -> ("error out"=w364:errorcluster, "Ctl Refnum"=w363:refnum<vi>, "uService Template out"=w365:refnum<class "Scheduler.lvclass">)  [unwired: 6 in]
          n134 = To More Specific Class(target class=w362, reference=w363, error in=w364) -> (specific class reference=w361:refnum<vi>, error out=w360:errorcluster)
          n135 = case shown="True" w377 {
            tunnel: w380 -> [_ w402]
            tunnel: w376 -> [_ w401]
            tunnel: w375 -> [_ w399]
            tunnel: [w387 w393] -> w370
            tunnel: w360 -> [w388 w395]
            tunnel: [TRUE ("Disable?") FALSE ("Disable?")] -> w371
            tunnel: w361 -> [w389 w394]
            frame False {
              n136 = invoke class="SubPnl" method="Remove VI"(reference=w389, error in=w388) -> (error out=w387:errorcluster)  [unwired: 1 in, 2 out]
            }
            frame True {
              n137 = Index Array(array=w402, index=w401) -> (element=w400:refnum<class "Sequence of SBlocks.lvclass">)
              n138 = call-dynamic "Get SBlock.vi"("error in (no error)"=w395, "index"=w399, "Sequence of SBlocks in"=w400) -> ("error out"=w397:errorcluster, "Schedule Block"=w398:refnum<class "Schedule Block.lvclass">)  [unwired: 6 in, 1 out]
              n139 = call-dynamic "Get GUI reference.vi"("error in (no error)"=w397, "Schedule Block in"=w398) -> ("error out"=w391:errorcluster, "This VI"=w392:refnum<vi>)  [unwired: 7 in, 1 out]
              n140 = invoke class="SubPnl" method="Insert VI"(reference=w394, error in=w391, "VI Ref"=w392) -> (error out=w393:errorcluster)  [unwired: 1 in, 3 out]
            }
          }
          n141 = call-dynamic "Disable Selection.vi"("error in (no error)"=w370, "Disable?"=w371, "Scheduler in"=w365) -> ("error out"=w372:errorcluster, "Scheduler out"=w373:refnum<class "Scheduler.lvclass">)  [unwired: 7 in]
          n142 = call "Substitute Error.vi"("LabVIEW Object"=w373, "error in (no error)"=w372, "Error Code"=5653) -> ("error out"=w386:errorcluster)  [unwired: 8 in]
        }
        frame "Load" {
          n143 = Variant To Data(error in=w413, type=refnum<file> refnum ("refnum out"), Variant=w414) -> (data=w420:refnum<file>, error out=w421:errorcluster)
          n144 = case shown="No Error" w421 {
            selector: w421 -> [w444 w464]
            tunnel: w416 -> [w434 w463]
            tunnel: [w443 w463] -> w417
            tunnel: w420 -> [w445 _]
            tunnel: [w430 w464] -> w419
            frame No Error {
              n145 = Read from Text File(file (use dialog)=w445, error in=w444) -> (refnum out=w440:refnum<file>, text=w437:string, error out=w441:errorcluster)  [unwired: 2 in, 1 out]
              n146 = Unflatten From XML(xml string=w437, type=refnum<class "Sequence of SBlocks.lvclass">[] [] ("Array of Seqs"), error in (no error)=w441) -> (value=w438:refnum<class "Sequence of SBlocks.lvclass">[], error out=w439:errorcluster)
              n147 = case shown="Error .." w439 {
                selector: w439 -> [w448 w456]
                tunnel: [w448 w449] -> w432
                tunnel: w438 -> [w447 _]
                tunnel: [w447 w450] -> w433
                tunnel: w437 -> [_ w455]
                frame No Error {
                }
                frame Error {
                  # "Error, maybe trying to read a file in the old format"
                  n148 = call <vilib>:"Clear Errors.vi"("error in (no error)"=w456) -> ("error out"=w454:errorcluster)  [unwired: 5 in, 1 out]
                  n149 = Unflatten From XML(xml string=w455, type=refnum<class "Schedule.lvclass"> refnum ("TALOS.lvlib:Run Utilities.lvlib:Schedule.lvclass"), error in (no error)=w454) -> (value=w451:refnum<class "Schedule.lvclass">, error out=w452:errorcluster)
                  n150 = case shown="Error .." w452 {
                    selector: w452 -> [_ w462]
                    tunnel: w451 -> [w460 _]
                    tunnel: [w458 refnum<class "Sequence of SBlocks.lvclass">[] []] -> w450
                    tunnel: [w457 w462] -> w449
                    frame No Error {
                      n151 = call "Convert Schedule to Sequence of SBlocks.vi"("Schedule"=w460) -> ("error out"=w457:errorcluster, "Sequence of SBlocks"=w459:refnum<class "Sequence of SBlocks.lvclass">)  [unwired: 1 in]
                      n152 = Build Array(w459) -> (w458:refnum<class "Sequence of SBlocks.lvclass">[])
                    }
                    frame Error {
                    }
                  }
                }
              }
              n153 = Close File(refnum=w440) -> (error out=w446:errorcluster)  [unwired: 1 in, 1 out]
              n154 = call-dynamic "Append Loaded Sequences.vi"("error in (no error)"=w432, "Array of Seqs Loaded"=w433, "Scheduler in"=w434) -> ("error out"=w431:errorcluster, "Scheduler out"=w435:refnum<class "Scheduler.lvclass">)  [unwired: 7 in]
              n155 = call-dynamic "Estimate Time.vi"("error in (no error)"=w431, "Scheduler in"=w435) -> ("error out"=w442:errorcluster, "Scheduler out"=w428:refnum<class "Scheduler.lvclass">)  [unwired: 8 in]
              n156 = call "Send to Consumer.vi"("error in (no error)"=w442, "Case ID"=Scheduler_Consumer_Case_Selector."Update GUI" ("Consumer Case Selector"), "uService Template in"=w428) -> ("error out"=w429:errorcluster, "uService Template out"=w443:refnum<class "Scheduler.lvclass">)  [unwired: 7 in]
              n157 = Merge Errors(w446, w429) -> (w430:errorcluster)
            }
            frame Error {
            }
          }
          n158 = case shown="Error .." w419 {
            selector: w419 -> [w422 w426]
            tunnel: [w422 w425] -> w418
            frame No Error {
            }
            frame Error {
              n159 = call <vilib>:"Clear Errors.vi"("error in (no error)"=w426) -> ("error out"=w423:errorcluster)  [unwired: 5 in, 1 out]
              n160 = call "Temporised Pop-up Window.vi"("error in (no error)"=w423, "Text"="Error while loading sequence from the file!") -> ("error out"=w425:errorcluster)  [unwired: 9 in]
            }
          }
        }
        frame "Save" {
          n161 = Variant To Data(error in=w466, type=refnum<file> refnum ("refnum out"), Variant=w467) -> (data=w472:refnum<file>, error out=w473:errorcluster)
          n162 = case shown="No Error" w473 {
            selector: w473 -> [w479 w489]
            tunnel: w468 -> [w484 w488]
            tunnel: [w484 w488] -> w469
            tunnel: w472 -> [w480 _]
            tunnel: [w486 w489] -> w471
            frame No Error {
              n163 = property class="Scheduler.lvclass"(reference=w484) -> ("Accessors:Array of Squences"=w481:refnum<class "Sequence of SBlocks.lvclass">[])  [unwired: 1 in, 2 out]
              n164 = Flatten To XML(6:w481) -> (2:w482:string)
              n165 = Write to Text File(file (use dialog)=w480, text=w482, error in=w479) -> (refnum out=w483:refnum<file>, error out=w485:errorcluster)  [unwired: 1 in, 1 out]
              n166 = Close File(refnum=w483) -> (error out=w487:errorcluster)  [unwired: 1 in, 1 out]
              n167 = Merge Errors(w487, w485) -> (w486:errorcluster)
            }
            frame Error {
            }
          }
          n168 = case shown="No Error" w471 {
            selector: w471 -> [w474 w478]
            tunnel: [w474 w477] -> w470
            frame No Error {
            }
            frame Error {
              n169 = call <vilib>:"Clear Errors.vi"("error in (no error)"=w478) -> ("error out"=w475:errorcluster)  [unwired: 5 in, 1 out]
              n170 = call "Temporised Pop-up Window.vi"("error in (no error)"=w475, "Text"="Error while saving the sequence in the file!") -> ("error out"=w477:errorcluster)  [unwired: 9 in]
            }
          }
        }
        frame "Duplicate SBlock" {
          n171 = Unbundle By Name(w496) -> ("Sequence Index"=w495:i32, "SBlock Index"=w494:i32)
          n172 = in-place {
            in-place-border: w497 -> [w502]
            in-place-border: w495 -> [w500]
            in-place-border: w494 -> [w499]
            in-place-border: [w498] -> w493
            n173 = in-place-cluster #9(w496) -> ("Array of Seqs"=w503:refnum<class "Sequence of SBlocks.lvclass">[])
            n174 = in-place {
              in-place-border: w499 -> [w507]
              in-place-border: w502 -> [w505]
              in-place-border: [w504] -> w498
              n175 = in-place-array #10(w503, w500) -> (w508:refnum<class "Sequence of SBlocks.lvclass">)
              n176 = call-dynamic "Duplicate SBlock.vi"("error in (no error)"=w505, "index"=w507, "Sequence of SBlocks in"=w508) -> ("error out"=w504:errorcluster, "Sequence of SBlocks out"=w506:refnum<class "Sequence of SBlocks.lvclass">)  [unwired: 7 in]
              n177 = in-place-array #10(w506) -> (w501:refnum<class "Sequence of SBlocks.lvclass">[])  [unwired: 1 out]
            }
            n178 = in-place-cluster #9("Array of Seqs"=w501) -> (w492:refnum<class "Scheduler.lvclass">)
          }
          n179 = call-dynamic "Estimate Time.vi"("error in (no error)"=w493, "Scheduler in"=w492) -> ("error out"=w490:errorcluster, "Scheduler out"=w491:refnum<class "Scheduler.lvclass">)  [unwired: 8 in]
        }
        frame "Select SBlock" {
          # "This is a programmer's error"
          # "#5659"
          n180 = Variant To Data(error in=w516, type=T8 {"Row"=-1, "Column"=-1}, Variant=w518) -> (data=w514:T8, error out=w510:errorcluster)
          n181 = Equal?(x=w514, y=cluster{i32, i32} {-1, -1}) -> (x = y?=w512:bool)
          n182 = call "Substitute Error.vi"("LabVIEW Object"=w519, "error in (no error)"=w510, "Error Code"=5659) -> ("error out"=w511:errorcluster)  [unwired: 8 in]
          n183 = case shown="False" w512 {
            tunnel: w519 -> [w522 w557]
            tunnel: [w521 w556] -> w515
            tunnel: w514 -> [w520 w555]
            frame False {
              n184 = in-place {
                in-place-border: w520 -> [w525]
                n185 = in-place-cluster #11(w522) -> ("Array of Seqs"=w529:refnum<class "Sequence of SBlocks.lvclass">[], "Sequence Index"=w527:i32, "SBlock Index"=w528:i32)
                n186 = Bundle("SBlock Index"=w528, "Sequence Index"=w527) -> (w526:T11)  [unwired: 1 in]
                n187 = Unbundle By Name(w525) -> ("Row"=w531:i32, "Column"=w532:i32)
                n188 = Equal?(x=w525, y=w526) -> (x = y?=w524:bool)
                n189 = case shown="False" w524 {
                  tunnel: w532 -> [w533 _]
                  tunnel: w527 -> [_ _]
                  tunnel: [w534 -1 ("Sequence Index")] -> w523
                  tunnel: w531 -> [w537 _]
                  tunnel: w529 -> [w536 _]
                  tunnel: [w535 -1 ("SBlock Index")] -> w530
                  frame False {
                    n190 = Array Size(array=w536) -> (size(s)=w539:i32)
                    n191 = Less Or Equal?(x=w539, y=w533) -> (x <= y?=w538:bool)
                    n192 = case shown="False" w538 {
                      tunnel: w536 -> [w549 _]
                      tunnel: w533 -> [w541 _]
                      tunnel: [w544 w550] -> w534
                      tunnel: w537 -> [w542 _]
                      tunnel: [w546 w550] -> w535
                      frame False {
                        # "Check if row is in range"
                        n193 = Index Array(array=w549, index=w541) -> (element=w548:refnum<class "Sequence of SBlocks.lvclass">)
                        n194 = call-dynamic "Get Size.vi"("Sequence of SBlocks in"=w548) -> ("size"=w547:i32)  [unwired: 8 in, 2 out]
                        n195 = Less Or Equal?(x=w547, y=w542) -> (x <= y?=w545:bool)
                        n196 = Select(t=-1 ("f"), s=w545, f=w541) -> (s? t:f=w544:i32)
                        n197 = Select(t=-1 ("f"), s=w545, f=w542) -> (s? t:f=w546:i32)
                      }
                      frame True {
                        w550 = -1 ("Row")
                        # "Index out of bounds"
                      }
                    }
                  }
                  frame True {
                  }
                }
                n198 = in-place-cluster #11("Array of Seqs"=w529, "Sequence Index"=w523, "SBlock Index"=w530) -> (w521:refnum<class "Scheduler.lvclass">)
              }
            }
            frame True {
              n199 = Unbundle(w555) -> ("Row"=w554:i32, "Column"=w553:i32)
              n200 = Bundle By Name(cluster=w557, "SBlock Index"=w554, "Sequence Index"=w553) -> (w556:refnum<class "Scheduler.lvclass">)
            }
          }
        }
        frame "Split/Combine Schedules" {
          # "#5660"
          n201 = property class="Scheduler.lvclass"(reference=w565) -> (reference out=w560:refnum<class "Scheduler.lvclass">, "Accessors:Array of Squences"=w559:refnum<class "Sequence of SBlocks.lvclass">[])  [unwired: 1 in, 1 out]
          n202 = Empty Array?(array=w559) -> (empty?=w558:bool)
          n203 = case shown="False" w558 {
            tunnel: w567 -> [w577 _]
            tunnel: w566 -> [w575 w587]
            tunnel: [w570 w586] -> w562
            tunnel: [w569 w587] -> w561
            tunnel: w560 -> [w568 w586]
            frame False {
              n204 = Variant To Data(error in=w575, type=FALSE, Variant=w577) -> (data=w574:bool, error out=w573:errorcluster)
              n205 = case shown="True" w574 {
                tunnel: w568 -> [w581 w585]
                tunnel: [w579 w583] -> w572
                tunnel: w573 -> [w580 w584]
                tunnel: [w578 w582] -> w571
                frame False {
                  # "Parallel mode off, combine all sequences into one"
                  n206 = call-dynamic "Concatenate Sequences.vi"("error in (no error)"=w580, "Scheduler in"=w581) -> ("error out"=w578:errorcluster, "Scheduler out"=w579:refnum<class "Scheduler.lvclass">)  [unwired: 8 in]
                }
                frame True {
                  # "Parallel mode on, split sequences into different columns"
                  n207 = call-dynamic "Split Sequences.vi"("error in (no error)"=w584, "Scheduler in"=w585) -> ("error out"=w582:errorcluster, "Scheduler out"=w583:refnum<class "Scheduler.lvclass">)  [unwired: 8 in]
                }
              }
              n208 = call-dynamic "Estimate Time.vi"("error in (no error)"=w571, "Scheduler in"=w572) -> ("error out"=w569:errorcluster, "Scheduler out"=w570:refnum<class "Scheduler.lvclass">)  [unwired: 8 in]
            }
            frame True {
              # "empty array, we are not doing anything"
            }
          }
          n209 = call "Substitute Error.vi"("LabVIEW Object"=w562, "error in (no error)"=w561, "Error Code"=5660) -> ("error out"=w564:errorcluster)  [unwired: 8 in]
        }
        frame "Reschedule" {
          n210 = Variant To Data(error in=w592, type=refnum<class "Sequence of SBlocks.lvclass"> refnum ("RSequence of SBlocks"), Variant=w597) -> (data=w594:refnum<class "Sequence of SBlocks.lvclass">, error out=w591:errorcluster)
          n211 = Build Array(w594) -> (w593:refnum<class "Sequence of SBlocks.lvclass">[])
          n212 = Bundle By Name(cluster=w595, "Array of Seqs"=w593) -> (w590:refnum<class "Scheduler.lvclass">)
          n213 = call-dynamic "Estimate Time.vi"("error in (no error)"=w591, "Scheduler in"=w590) -> ("error out"=w588:errorcluster, "Scheduler out"=w589:refnum<class "Scheduler.lvclass">)  [unwired: 8 in]
        }
        frame "Load Parameters" {
          n214 = call-dynamic "Load Parameters.vi"("error in (no error)"=w601, "Scheduler in"=w600) -> ("error out"=w598:errorcluster, "Scheduler out"=w599:refnum<class "Scheduler.lvclass">)  [unwired: 8 in]
        }
      }
    }
    frame Error {
    }
  }
  n215 = call-parent "Consumer.vi"("error in (no error)"=w6, "Data"="Data", "Case ID"="Case ID", "uService Template in"=w3) -> ("error out"=→"error out":errorcluster, "uService Template out"=→"Scheduler out":refnum<class "Scheduler.lvclass">)  [unwired: 6 in]
